vi "HoldingRegisters.vi"(0 "Handle In":u64[](array[numeric]), 1 "Device ID":u8=1, 2 "Read Start":u16=17, 3 "Read Amount":u16=16, 4 "Write Start":u16=1, 5 "Write Amount":u16=16, 6 "WR Data":u16[](array[numeric]), 7 "Operation":T1(ring), 8 "error in (no error)":errorcluster) -> (18 "error out":errorcluster, 20 "Handle Out":u64[](array[numeric]), 21 "Result":i32, 22 "RD/WR Data":u16[](array[numeric]))   [LabVIEW 2020, in "SnapMB.lvlib"]
uses:
  SnapMB.lvlib
  windows/snapmb.dll
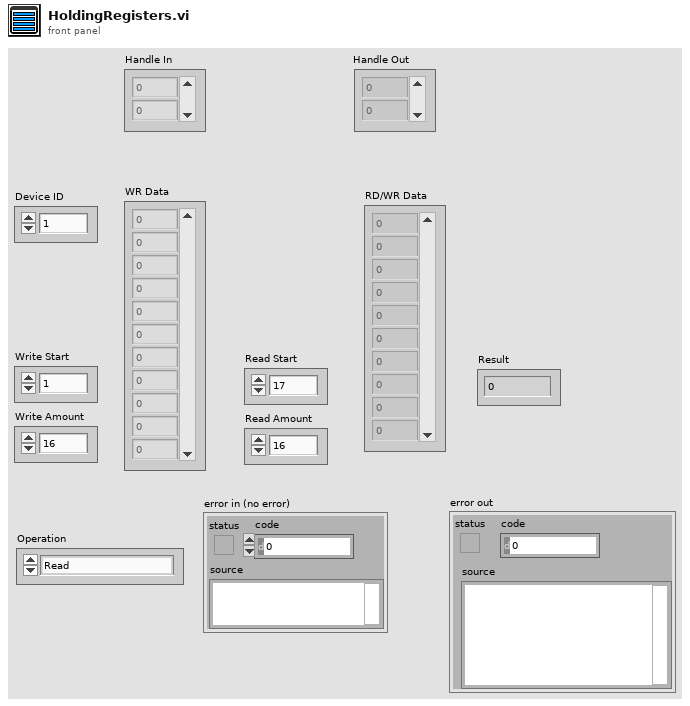
[diagram p1: front panel]
types:
  T1 = enum16{"Read", "Write", "Read/Write (Fun 0x17)", "Read/Write (Sequential)"}
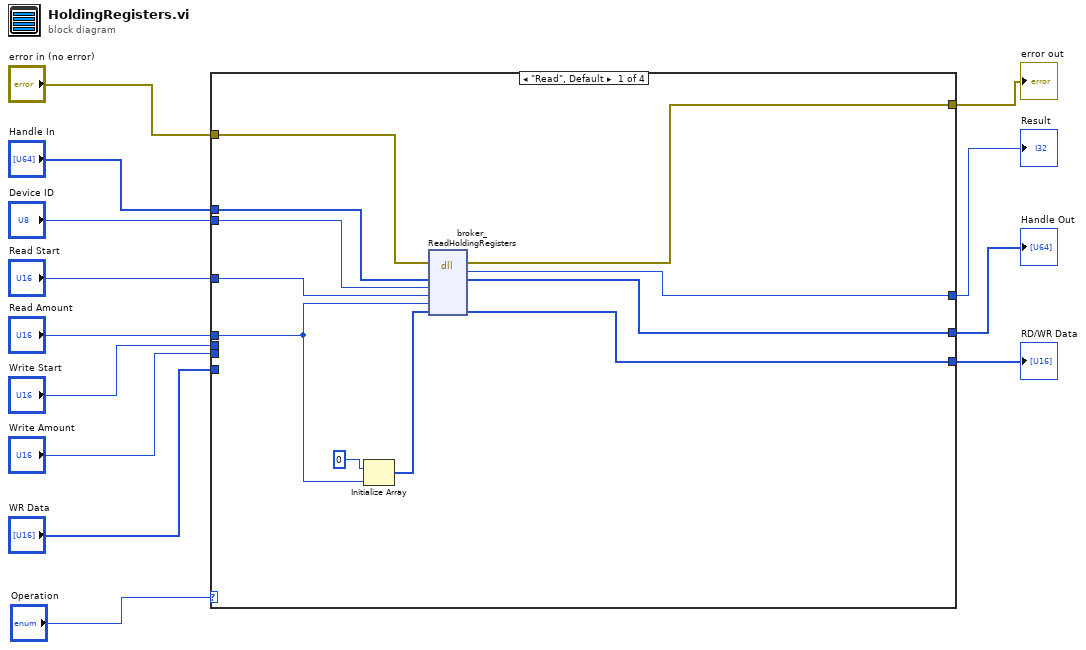
[diagram p0: block diagram]
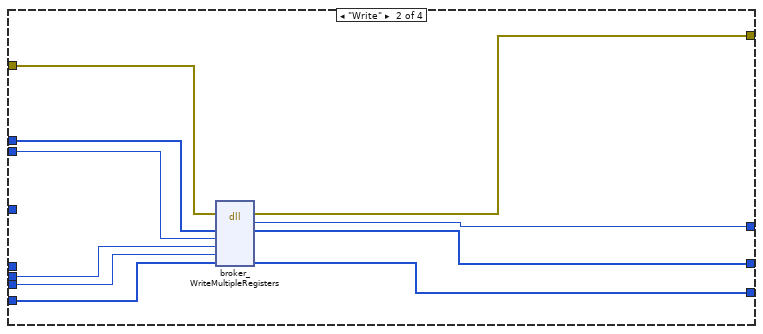
[diagram p2: hidden frame]
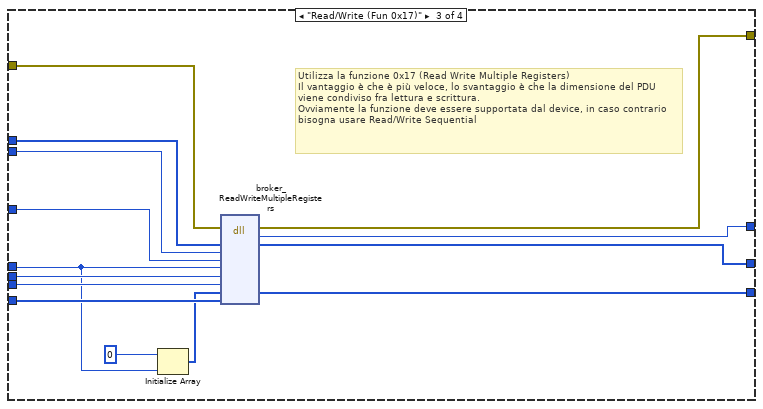
[diagram p3: hidden frame]
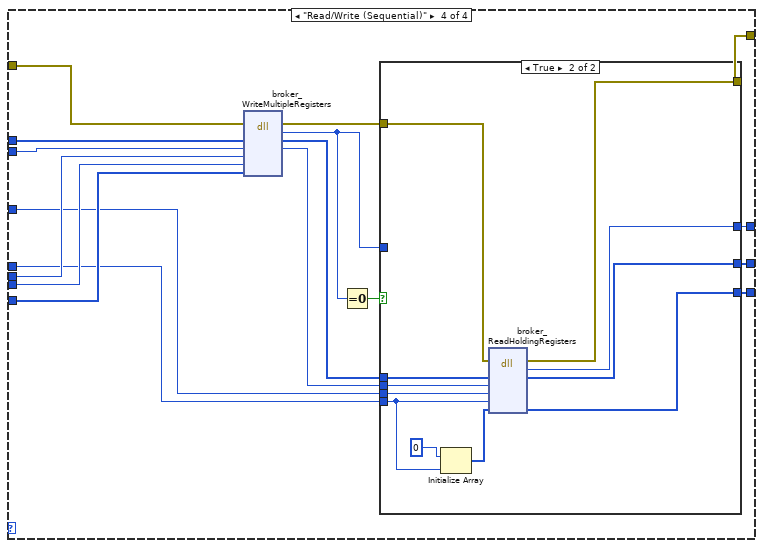
[diagram p4: hidden frame]
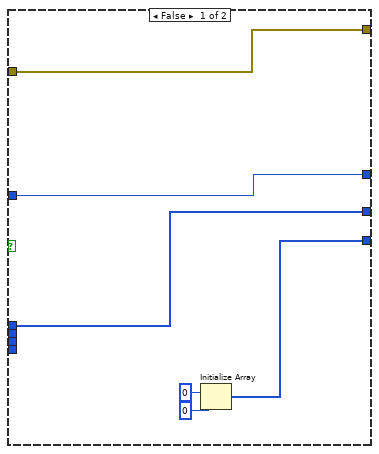
[diagram p5: hidden frame]
diagram:
  n1 = case shown="\"Read\", Default" "Operation" {
    tunnel: "Handle In" -> [w19 w33 w48 w61]
    tunnel: "Device ID" -> [w20 w32 w47 w60]
    tunnel: "Read Start" -> [w21 _ w46 w54]
    tunnel: "Read Amount" -> [w22 _ w38 w53]
    tunnel: "Write Start" -> [_ w31 w45 w65]
    tunnel: "Write Amount" -> [_ w30 w44 w64]
    tunnel: "WR Data" -> [_ w29 w43 w63]
    tunnel: [w18 w25 w42 w57] -> w5
    tunnel: [w17 w28 w41 w59] -> w4
    tunnel: [w14 w27 w36 w55] -> w3
    tunnel: "error in (no error)" -> [w16 w34 w40 w51]
    tunnel: [w15 w26 w35 w50] -> w1
    frame "Read", Default {
      n2 = Initialize Array(u16 0 ("element"), w22) -> (w23:u16[])
      n3 = dll-call lib="D:/SnapMB/LabView/lib/windows/snapmb.dll" fn="broker_ReadHoldingRegisters"(error in=w16, "Handle"=w19, "DeviceID"=w20, "Start"=w21, "Amount"=w22, "pUsrData"=w23) -> (error out=w15:errorcluster, "Result"=w17:i32, "Handle"=w14:u64[], "pUsrData"=w18:u16[])  [unwired: 5 in, 1 out]
    }
    frame "Write" {
      n4 = dll-call lib="D:/SnapMB/LabView/lib/windows/snapmb.dll" fn="broker_WriteMultipleRegisters"(error in=w34, "Handle"=w33, "DeviceID"=w32, "Start"=w31, "Amount"=w30, "pUsrData"=w29) -> (error out=w26:errorcluster, "Result"=w28:i32, "Handle"=w27:u64[], "pUsrData"=w25:u16[])  [unwired: 5 in, 1 out]
    }
    frame "Read/Write (Fun 0x17)" {
      # "Utilizza la funzione 0x17 (Read Write Multiple Registers)\nIl vantaggio è che è più veloce, lo svantaggio è che la dimensione del PDU viene condiviso fra lettura e scrittura.\nOvviamente la funzione deve essere supportata dal device, in caso contrario bisogna usare Read/Write Sequential"
      n5 = Initialize Array(u16 0 ("element"), w38) -> (w37:u16[])
      n6 = dll-call lib="D:/SnapMB/LabView/lib/windows/snapmb.dll" fn="broker_ReadWriteMultipleRegisters"(error in=w40, "Handle"=w48, "DeviceID"=w47, "RDStart"=w46, "RDAmount"=w38, "WRStart"=w45, "WRAmount"=w44, "RDUsrData"=w37, "WRUsrData"=w43) -> (error out=w35:errorcluster, "Result"=w41:i32, "Handle"=w36:u64[], "RDUsrData"=w42:u16[])  [unwired: 8 in, 1 out]
    }
    frame "Read/Write (Sequential)" {
      n7 = dll-call lib="D:/SnapMB/LabView/lib/windows/snapmb.dll" fn="broker_WriteMultipleRegisters"(error in=w51, "Handle"=w61, "DeviceID"=w60, "Start"=w65, "Amount"=w64, "pUsrData"=w63) -> (error out=w49:errorcluster, "Result"=w58:i32, "Handle"=w56:u64[], "DeviceID"=w52:u8)  [unwired: 5 in, 1 out]
      n8 = Equal To 0?(x=w58) -> (x = 0?=w62:bool)
      n9 = case shown="True" w62 {
        tunnel: [w70 w82] -> w59
        tunnel: w58 -> [w70 _]
        tunnel: [w67 w81] -> w57
        tunnel: w56 -> [w71 w80]
        tunnel: [w71 w79] -> w55
        tunnel: w54 -> [_ w76]
        tunnel: w53 -> [_ w74]
        tunnel: w52 -> [_ w75]
        tunnel: [w66 w73] -> w50
        tunnel: w49 -> [w66 w72]
        frame False {
          n10 = Initialize Array(u16 0 ("element"), 0 ("dimension size")) -> (w67:u16[])
        }
        frame True {
          n11 = Initialize Array(u16 0 ("element"), w74) -> (w77:u16[])
          n12 = dll-call lib="D:/SnapMB/LabView/lib/windows/snapmb.dll" fn="broker_ReadHoldingRegisters"(error in=w72, "Handle"=w80, "DeviceID"=w75, "Start"=w76, "Amount"=w74, "pUsrData"=w77) -> (error out=w73:errorcluster, "Result"=w82:i32, "Handle"=w79:u64[], "pUsrData"=w81:u16[])  [unwired: 5 in, 1 out]
        }
      }
    }
  }
  "Result" <- w4
  "RD/WR Data" <- w5
  "Handle Out" <- w3
  "error out" <- w1
